vi "send_AMKActualValues.vi"(4 "Counter":i32, 5 "200/freq":i32=1, 6 "Active":bool, 7 "CAN ID":u32=644 format="%x", 8 "Message":T1 {"AMK_ActualVelocity" scale=0.0..21500.0}, 11 "CAN frame":T2[](array[typedef]) {"Data" format="%.0x"; "ArbitrationId" format="%.0x"; "Timestamp" format="%<%I:%M:%S%3u %p\n%m/%d/%Y>T"}) -> (3 "CAN frame out":T2[](array[typedef]) {"Data" format="%.0x"; "ArbitrationId" format="%.0x"; "Timestamp" format="%<%I:%M:%S%3u %p\n%m/%d/%Y>T"})   [LabVIEW 2017]
uses:
  <vilib>/nican/nican.llb/CanFrameTimed.ctl
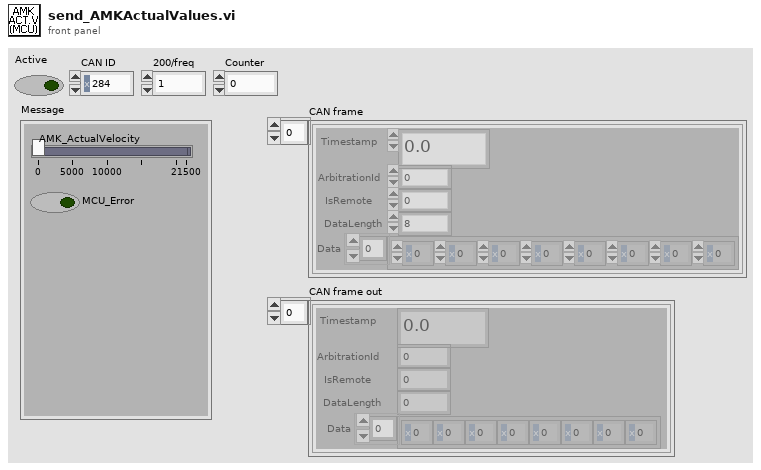
[diagram p1: front panel]
types:
  T1 = cluster{"MCU_Error":bool, "AMK_ActualVelocity":dbl}
  T2 = typedef "CanFrameTimed.ctl" = cluster{"Timestamp":dbl, "ArbitrationId":u32, "IsRemote":u8, "DataLength":u8, "Data":u8[]}
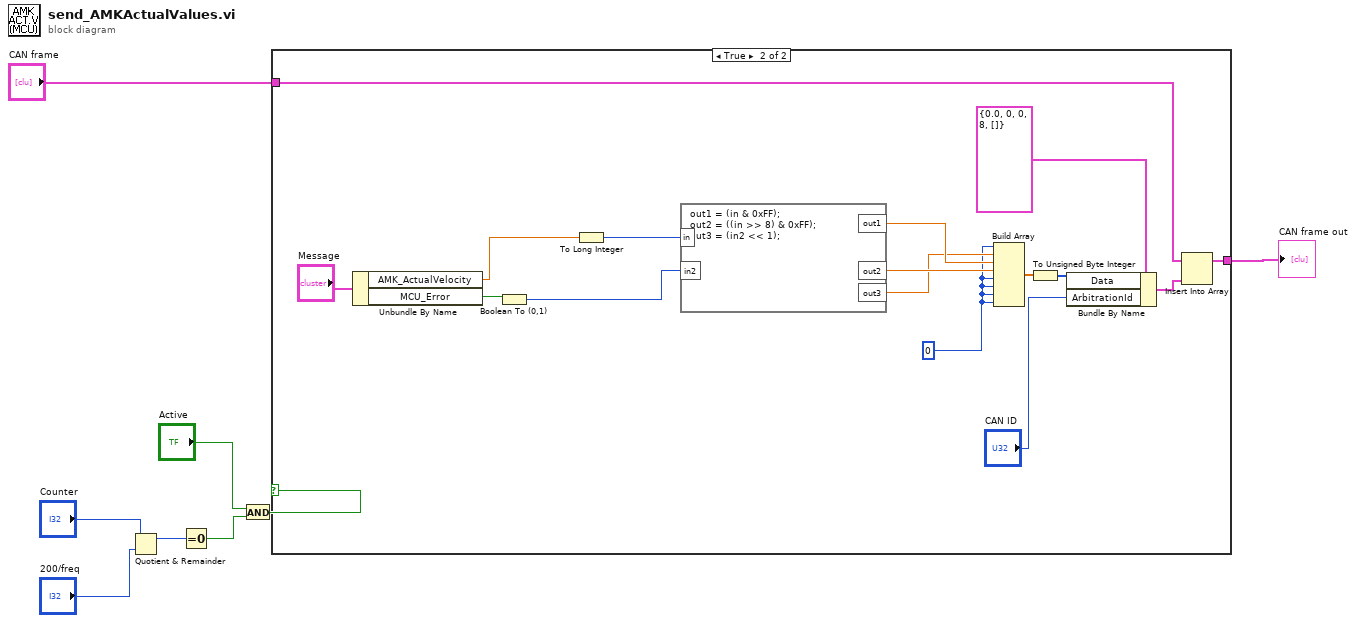
[diagram p0: block diagram]
diagram:
  n1 = Quotient & Remainder(x="Counter", y="200/freq") -> (x-y*floor(x/y)=w5:i32)  [unwired: 1 out]
  n2 = Equal To 0?(x=w5) -> (x = 0?=w3:bool)
  n3 = And(x="Active", y=w3) -> (x .and. y?=w2:bool)
  n4 = case shown="True" w2 {
    tunnel: "CAN frame" -> [w9 w22]
    tunnel: [w9 w20] -> w7
    frame False {
    }
    frame True {
      w13 = u8 0 ("Byte 0")
      n5 = Unbundle By Name("Message") -> ("AMK_ActualVelocity"=w11:dbl, "MCU_Error"=w12:bool)
      n6 = Boolean To (0,1)(Boolean=w12) -> (0, 1=w18:i16)
      n7 = To Long Integer(number=w11) -> (32bit integer=w10:i32)
      n8 = formula code="out1 = (in & 0xFF);\nout2 = ((in >> 8) & 0xFF);\nout3 = (in2 << 1);"("in"=w10, "in2"=w18) -> ("out1"=w15:dbl, "out2"=w16:dbl, "out3"=w14:dbl)
      n9 = Build Array(w13, w14, w15, w16, w13, w13, w13, w13) -> (w25:dbl[])
      n10 = To Unsigned Byte Integer(number=w25) -> (unsigned 8bit integer=w24:u8[])
      n11 = Bundle By Name(cluster=T2 {"Timestamp"=0.0, "ArbitrationId"=0, "IsRemote"=0, "DataLength"=8, "Data"=[]} ("CAN frame"), "Data"=w24, "ArbitrationId"="CAN ID") -> (w21:T2)
      n12 = Insert Into Array(array=w22, new element=w21) -> (w20:T2[])  [unwired: 1 in]
    }
  }
  "CAN frame out" <- w7
